vi "Launch Series.vi"(8 "error in":errorcluster, 11 "Configuration UI Actor in":refnum<class "Configuration UI Actor.lvclass">) -> (0 "error out":errorcluster, 3 "Configuration UI Actor out":refnum<class "Configuration UI Actor.lvclass">)   [LabVIEW 2023, in "Configuration UI Actor.lvlib" / "Configuration UI Actor.lvclass"]
uses:
  Configuration UI Actor.lvclass
  Configuration UI Actor.lvclass/Configuration UI Actor.ctl
  <vilib>/ActorFramework/Actor/Actor.lvclass
  gitlab/imponator-actor/IMain Actor/IMain Actor Messages/Launch Series Msg/Launch Series Msg.lvclass
  C:/Program Files/National Instruments/LabVIEW 2023/vi.lib/MGI/Panel Manager/Panel Actor/Panel Actor/Panel Actor.lvclass
  C:/Program Files/National Instruments/LabVIEW 2023/vi.lib/ActorFramework/Actor/Actor.lvclass
  D:/git/HAL/Configurator/Configuration UI Actor/Configuration UI Actor.lvclass
  D:/git/HAL/Configurator/IConfiguration UI Actor/IConfiguration UI Actor/IConfiguration UI Actor.lvclass
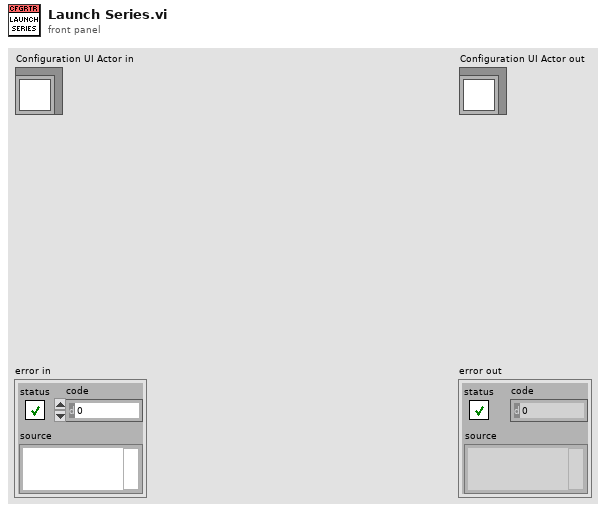
[diagram p1: front panel]
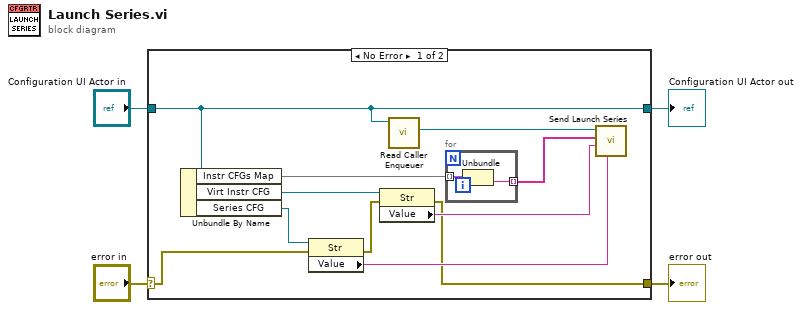
[diagram p0: block diagram]
diagram:
  n1 = case shown="No Error" "error in" {
    selector: "error in" -> [w7 w19]
    tunnel: [w5 w19] -> w3
    tunnel: [w15 w18] -> w1
    tunnel: "Configuration UI Actor in" -> [w15 w18]
    frame No Error {
      n2 = Unbundle By Name(w15) -> ("Instr CFGs Map"=w12:map{string, string}, "Virt Instr CFG"=w14:refnum<vi>, "Series CFG"=w13:refnum<vi>)
      n3 = property class="Str"(reference=w13, error in=w7) -> (error out=w6:errorcluster, "Value"=w8:string)  [unwired: 1 out]
      n4 = property class="Str"(reference=w14, error in=w6) -> (error out=w5:errorcluster, "Value"=w9:string)  [unwired: 1 out]
      n5 = call <vilib>:"Read Caller Enqueuer.vi"("Actor"=w15) -> ("Caller Enqueuer"=w11:refnum<class "Message Enqueuer.lvclass">)  [unwired: 10 in]
      n6 = for {
        tunnel: w12 -> [w17] mode=indexing
        tunnel: [w16] -> w10 mode=indexing
        n7 = Unbundle(w17) -> ("Instr Configuration"=w16:string)  [unwired: 1 out]
      }
      n8 = call "Send Launch Series.vi"("Series CFG"=w8, "Virt Instrs CFG"=w9, "Instr CFGS"=w10, "Message Enqueuer"=w11) -> ()  [unwired: 6 in, 2 out]
    }
    frame Error {
    }
  }
  "error out" <- w3
  "Configuration UI Actor out" <- w1
